vi "_Refresh Module By Name.vi"(8 "error in":errorcluster, 11 "Module Name":string) -> (0 "error out":errorcluster)   [LabVIEW 2020, in "Panther Dasboard Scripting Hooks.lvlib"]
uses:
  Panther Dasboard Scripting Hooks.lvlib
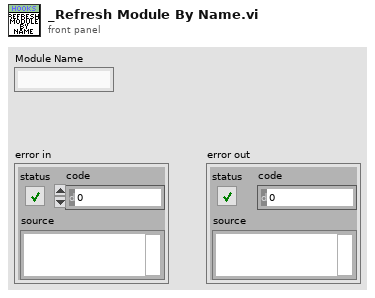
[diagram p1: front panel]
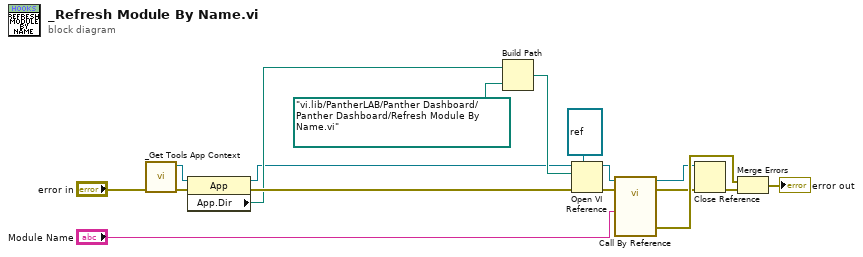
[diagram p0: block diagram]
diagram:
  n1 = call "_Get Tools App Context.vi"("error in"="error in") -> ("error out"=w11:errorcluster, "Application Context"=w2:refnum<vi>)  [unwired: 9 in]
  n2 = property class="App"(reference=w2, error in=w11) -> (reference out=w1:refnum<vi>, error out=w12:errorcluster, "App.Dir"=w5:path)
  n3 = Build Path(base path=w5, name or relative path=path "vi.lib/PantherLAB/Panther Dashboard/Panther Dashboard/Refresh Module By Name.vi") -> (appended path=w7:path)
  n4 = Open VI Reference(type specifier VI Refnum (for type only)=refnum<vi> refnum, application reference (local)=w1, vi path=w7, error in (no error)=w12) -> (vi reference=w8:refnum<vi>, error out=w13:errorcluster)  [unwired: 2 in]
  n5 = call-by-ref "?"(reference=w8, error in=w13, "Module Name"="Module Name") -> (reference out=w9:refnum<vi>, error out=w14:errorcluster, 0:"error out"=w17:errorcluster)  [unwired: 10 in]
  n6 = Close Reference(reference=w9, error in (no error)=w14) -> (error out=w15:errorcluster)
  n7 = Merge Errors(w17, w15) -> (→"error out":errorcluster)
